vi "Check .NET Objects Equal.vi"(8 "error in":errorcluster, 10 "object 2":refnum<k24>, 11 "object 1":refnum<k24>) -> (0 "error out":errorcluster, 3 "Equal?":bool)   [LabVIEW 2017, in "SLSC Switch Import Export Unit Tests.lvclass"]
uses:
  SLSC Switch Import Export Unit Tests.lvclass
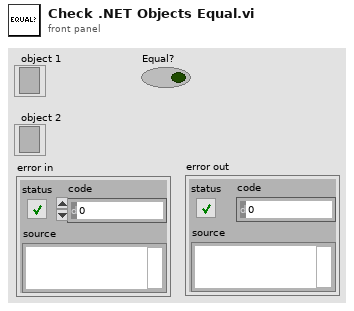
[diagram p1: front panel]
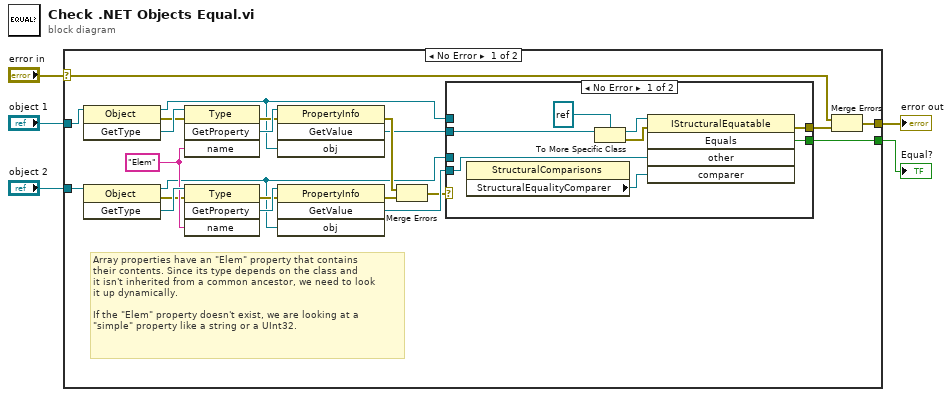
[diagram p0: block diagram]
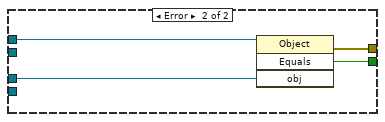
[diagram p2: hidden frame]
diagram:
  n1 = case shown="No Error" "error in" {
    selector: "error in" -> [w17 w40]
    tunnel: [w27 _] -> w5
    tunnel: "object 2" -> [w26 _]
    tunnel: "object 1" -> [w20 _]
    tunnel: [w15 w40] -> w1
    frame No Error {
      w21 = "Elem" ("name")
      # "Array properties have an \"Elem\" property that contains\ntheir contents. Since its type depends on the class and\nit isn't inherited from a common ancestor, we need to look\nit up dynamically.\n\nIf the \"Elem\" property doesn't exist, we are looking at a \n\"simple\" property like a string or a UInt32."
      n2 = invoke class="Object" method="GetType"(reference=w20) -> (reference out=w7:refnum<k24>, error out=w19:errorcluster, "GetType"=w25:refnum<k24>)  [unwired: 2 in]
      n3 = invoke class="Object" method="GetType"(reference=w26) -> (reference out=w6:refnum<k24>, error out=w18:errorcluster, "GetType"=w24:refnum<k24>)  [unwired: 2 in]
      n4 = invoke class="Type" method="GetProperty"(reference=w25, error in=w19, "name"=w21) -> (error out=w14:errorcluster, "GetProperty"=w22:refnum<k24>)  [unwired: 1 in, 2 out]
      n5 = invoke class="Type" method="GetProperty"(reference=w24, error in=w18, "name"=w21) -> (error out=w13:errorcluster, "GetProperty"=w23:refnum<k24>)  [unwired: 1 in, 2 out]
      n6 = invoke class="PropertyInfo" method="GetValue"(reference=w22, error in=w14, "obj"=w7) -> (error out=w10:errorcluster, "GetValue"=w8:refnum<k24>)  [unwired: 1 in, 2 out]
      n7 = invoke class="PropertyInfo" method="GetValue"(reference=w23, error in=w13, "obj"=w6) -> (error out=w11:errorcluster, "GetValue"=w12:refnum<k24>)  [unwired: 1 in, 2 out]
      n8 = Merge Errors(w10, w11) -> (w9:errorcluster)
      n9 = case shown="No Error" w9 {
        tunnel: [w35 w39] -> w27
        tunnel: [w34 w38] -> w16
        tunnel: w12 -> [w33 _]
        tunnel: w8 -> [w29 _]
        tunnel: w7 -> [_ w37]
        tunnel: w6 -> [_ w36]
        frame No Error {
          n10 = property class="StructuralComparisons"() -> ("StructuralEqualityComparer"=w28:refnum<k24>)  [unwired: 2 in, 2 out]
          n11 = To More Specific Class(target class=refnum<k24> refnum ("reference"), reference=w29) -> (specific class reference=w32:refnum<k24>, error out=w30:errorcluster)  [unwired: 1 in]
          n12 = invoke class="IStructuralEquatable" method="Equals"(reference=w32, error in=w30, "other"=w33, "comparer"=w28) -> (error out=w34:errorcluster, "Equals"=w35:bool)  [unwired: 1 in, 3 out]
        }
        frame Error {
          n13 = invoke class="Object" method="Equals"(reference=w37, "obj"=w36) -> (error out=w38:errorcluster, "Equals"=w39:bool)  [unwired: 2 in, 2 out]
        }
      }
      n14 = Merge Errors(w17, w16) -> (w15:errorcluster)
    }
    frame Error {
    }
  }
  "Equal?" <- w5
  "error out" <- w1
